vi "SRV_Append Line to File.vi"(0 "file path":path, 5 "Line to Write":string, 11 "error in (no error)":errorcluster) -> (15 "error out":errorcluster)   [LabVIEW 2009]
doc: "This VI appends \"Line to Write\" to the end of an existing file or creates a new one if necessary. It then writes an EOL to the end of the file.\n\nIt also sets the accesss rights of the file to read/write.\n\n\nAuthor: Mike Schultz"
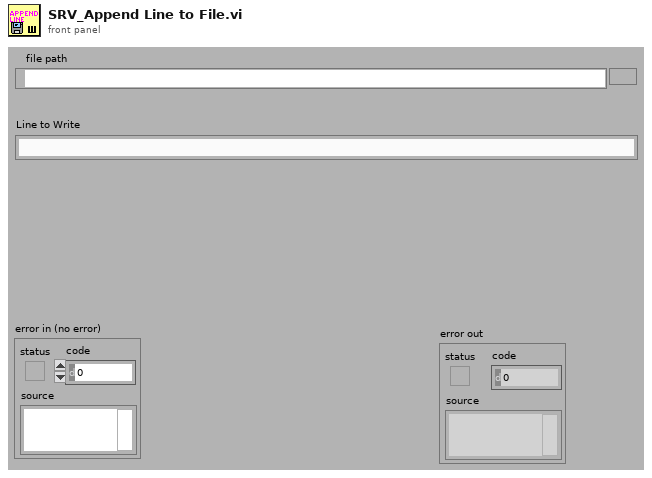
[diagram p1: front panel]
types:
  T1 = enum16{"open", "open or create", "create or replace", "create", "open (read only)"}
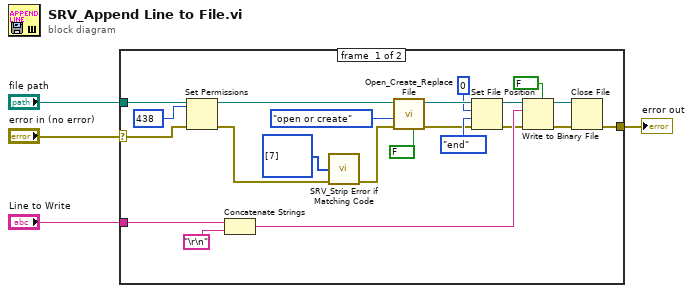
[diagram p0: block diagram]
diagram:
  n1 = case shown="No Error" "error in (no error)" {
    selector: "error in (no error)" -> [w9 w27]
    tunnel: "Line to Write" -> [w25 _]
    tunnel: [w21 w27] -> w3
    tunnel: "file path" -> [w15 _]
    frame #0 {
      n2 = Set Permissions(7:i16 438 ("new permissions"), 8:w9, 11:w15) -> (0:w12:errorcluster, 3:w14:path)  [unwired: 2 out]
      n3 = Concatenate Strings(w25, "\r\n") -> (w24:string)
      n4 = call "SRV_Strip Error if Matching Code.vi"("error in (no error)"=w12, "Strip Codes"=i32[] [7]) -> ("error out"=w13:errorcluster)  [unwired: 8 in]
      n5 = call <vilib>:"Open_Create_Replace File.vi"("advisory dialog? (display:T)"=FALSE, "error in (no error)"=w13, "function (open:0)"=T1."open or create", "file path"=w14) -> ("error out"=w11:errorcluster, "refnum"=w20:refnum<file>)  [unwired: 3 in, 3 out]
      n6 = Set File Position(offset (in bytes) (0)=i64 0, refnum=w20, from (0:start)=enum16{"start", "end", "current"}."end" ("pos mode (0:2)"), error in=w11) -> (refnum out=w8:refnum<file>, error out=w7:errorcluster)
      n7 = Write to Binary File(file (use dialog)=w8, data=w24, error in=w7, 5:FALSE ("prepend array or string size? (T)")) -> (refnum out=w22:refnum<file>, error out=w23:errorcluster)  [unwired: 3 out]
      n8 = Close File(refnum=w22, error in=w23) -> (error out=w21:errorcluster)  [unwired: 1 out]
    }
    frame #1 {
    }
  }
  "error out" <- w3
